vi "exponential curve fitting2015.vi"() -> ()   [LabVIEW 2015]
uses:
  <vilib>/Analysis/NI_AALPro.lvlib
  <vilib>/Utility/file.llb/Read Delimited Spreadsheet (DBL).vi
panel:
  out "Prepared by \nthe project":string
  in  "Measurement file \nwith extension Txt":path
  out "Data":dbl[][](array[numeric])
  out "Exponential Curve Fitting":dbl[](graph)
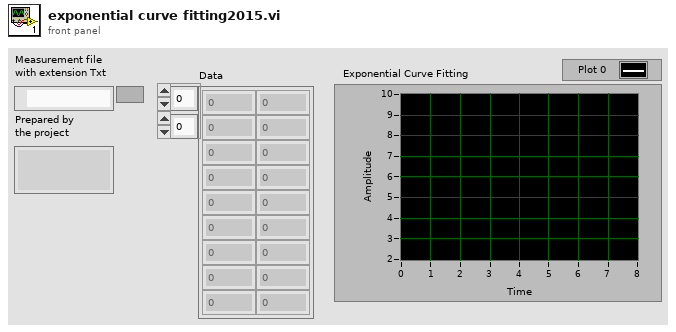
[diagram p1: front panel]
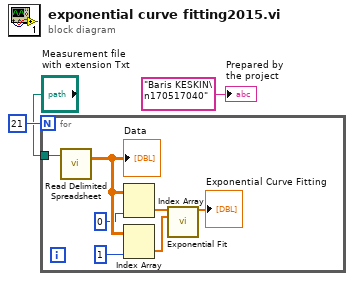
[diagram p0: block diagram]
diagram:
  n1 = for {
    N: 21 -> [_]
    tunnel: "Measurement file \nwith extension Txt" -> [w7]
    n2 = call-poly <vilib>:"Read Delimited Spreadsheet.vi"("file path (dialog if empty)"=w7) -> ("all rows"=w10:dbl[][])  [unwired: 9 in, 5 out]
    "Data" <- w10
    n3 = Index Array(array=w10, index (col)=0 ("disabled index (col)")) -> (element=w6:dbl[])  [unwired: 1 in]
    n4 = Index Array(array=w10, index (col)=1 ("disabled index (col)")) -> (element=w5:dbl[])  [unwired: 1 in]
    n5 = call <vilib>:"Exponential Fit.vi"("Y"=w6, "X"=w5) -> ("Best Exponential Fit"=→"Exponential Curve Fitting":dbl[])  [unwired: 8 in, 5 out]
  }
  "Prepared by \nthe project" <- "Baris KESKIN\n170517040"
